vi "sub vi - Read Analog All v9.5.vi"(0 "data 0":waveform(dbl)[](array[waveform]), 5 "data 1":waveform(dbl)[](array[waveform]), 7 "data 2":waveform(dbl)[](array[waveform]), 9 "AI Error":errorcluster[](array[cluster])) -> (3 "array GRAPH":dynamicdata[](array[waveform]), 4 "LAB01":T2, 6 "LAB02":T3, 8 "LAB03":T4, 10 "LAB04":T5, 13 "deg C":dbl, 14 "USB Error":bool[](array[boolean]), 15 "LAB05":T6)   [LabVIEW 2013]
uses:
  program files/Global display 3.vi
  <vilib>/measure/mascope.llb/Amplitude and Levels 1 chan.vi
  <vilib>/addons/Electrical Power/Basic/Measurement/Power (1 Channel).vi
  <vilib>/addons/Electrical Power/Basic/Measurement/RMS (N Channels).vi
  <vilib>/addons/Electrical Power/Basic/Measurement/RMS (1 Channel).vi
  <vilib>/addons/Electrical Power/Basic/NI_EP_Basic.lvlib
  <vilib>/measure/NI_MAPro.lvlib
panel:
  in  "Tab Control":T1(tab)
  out "LAB01-2 (PF)":dbl
  out "LAB01-1 (PF)":dbl
  out "LAB01-2 (V)":dbl
  out "LAB01-2 (A)":dbl
  out "LAB01-1 (V)":dbl
  out "LAB01-1 (A)":dbl
  out "LAB01-2 (GRAPH)":dynamicdata(graph)
  out "LAB01-1 (GRAPH)":dynamicdata(graph)
  out "LAB02-2 (PF)":dbl
  out "LAB02-1 (PF)":dbl
  out "LAB02-2 (V)":dbl
  out "LAB02-2 (A)":dbl
  out "LAB02-1 (V)":dbl
  out "LAB02-1 (A)":dbl
  out "LAB02-2 (GRAPH)":dynamicdata(graph)
  out "LAB02-1 (GRAPH)":dynamicdata(graph)
  out "LAB03-2 (PF)":dbl
  out "LAB03-1 (PF)":dbl
  out "LAB03-2 (V)":dbl
  out "LAB03-2 (A)":dbl
  out "LAB03-1 (V)":dbl
  out "LAB03-1 (A)":dbl
  out "LAB03-2 (GRAPH)":dynamicdata(graph)
  out "LAB03-1 (GRAPH)":dynamicdata(graph)
  out "LAB04-2 (PF)":dbl
  out "LAB04-1 (PF)":dbl
  out "LAB04-2 (V)":dbl
  out "LAB04-2 (A)":dbl
  out "LAB04-1 (V)":dbl
  out "LAB04-1 (A)":dbl
  out "LAB04-1 (GRAPH)":dynamicdata(graph)
  out "LAB04-2 (GRAPH)":dynamicdata(graph)
  out "LAB05-2 (PF)":dbl
  out "LAB05-1 (PF)":dbl
  out "LAB05-2 (V)":dbl
  out "LAB05-2 (A)":dbl
  out "LAB05-1 (V)":dbl
  out "LAB05-1 (A)":dbl
  out "LAB05-1 (GRAPH)":dynamicdata(graph)
  out "LAB05-2 (GRAPH)":dynamicdata(graph)
  out "A1 error":errorcluster
  out "array ERROR":errorcluster[](array[cluster])
  out "AI2-OFF":waveform(dbl)[](graph)
  out "AI2-ON":waveform(dbl)[](graph)
  out "AI1-OFF":waveform(dbl)[](graph)
  out "AI1-ON":waveform(dbl)[](graph)
  out "AI0-OFF":waveform(dbl)[](graph)
  out "AI0-ON":waveform(dbl)[](graph)
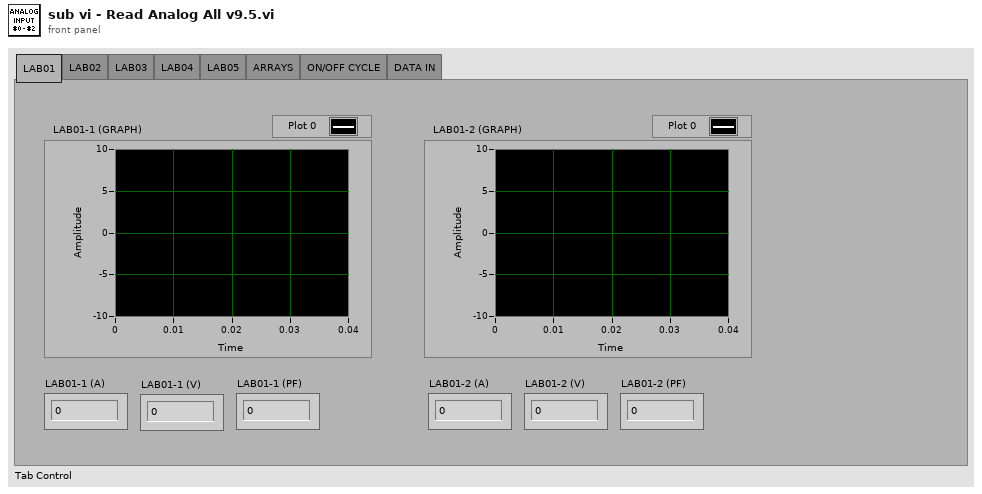
[diagram p1: front panel]
types:
  T1 = enum32{"LAB01", "LAB02", "LAB03", "LAB04", "LAB05", "ARRAYS", "ON/OFF CYCLE", "DATA IN"}
  T2 = cluster{"LAB01-1 (A)":dbl, "LAB01-1 (V)":dbl, "LAB01-1 (PF)":dbl, "LAB01-2 (A)":dbl, "LAB01-2 (V)":dbl, "LAB01-2 (PF)":dbl}
  T3 = cluster{"LAB02-1 (A)":dbl, "LAB02-1 (V)":dbl, "LAB02-1 (PF)":dbl, "LAB02-2 (A)":dbl, "LAB02-2 (V)":dbl, "LAB02-2 (PF)":dbl}
  T4 = cluster{"LAB03-1 (A)":dbl, "LAB03-1 (V)":dbl, "LAB03-1 (PF)":dbl, "LAB03-2 (A)":dbl, "LAB03-2 (V)":dbl, "LAB03-2 (PF)":dbl}
  T5 = cluster{"LAB04-1 (A)":dbl, "LAB04-1 (V)":dbl, "LAB04-1 (PF)":dbl, "LAB04-2 (A)":dbl, "LAB04-2 (V)":dbl, "LAB04-2 (PF)":dbl}
  T6 = cluster{"LAB05-1 (A)":dbl, "LAB05-1 (V)":dbl, "LAB05-1 (PF)":dbl, "LAB05-2 (A)":dbl, "LAB05-2 (V)":dbl, "LAB05-2 (PF)":dbl}
  T7 = typedef "NI_EP_Basic.lvlib/basic_Power Value.ctl" = cluster{"active power [W]":dbl, "apparent power [VA]":dbl, "reactive power [VAR]":dbl, "power factor":dbl}
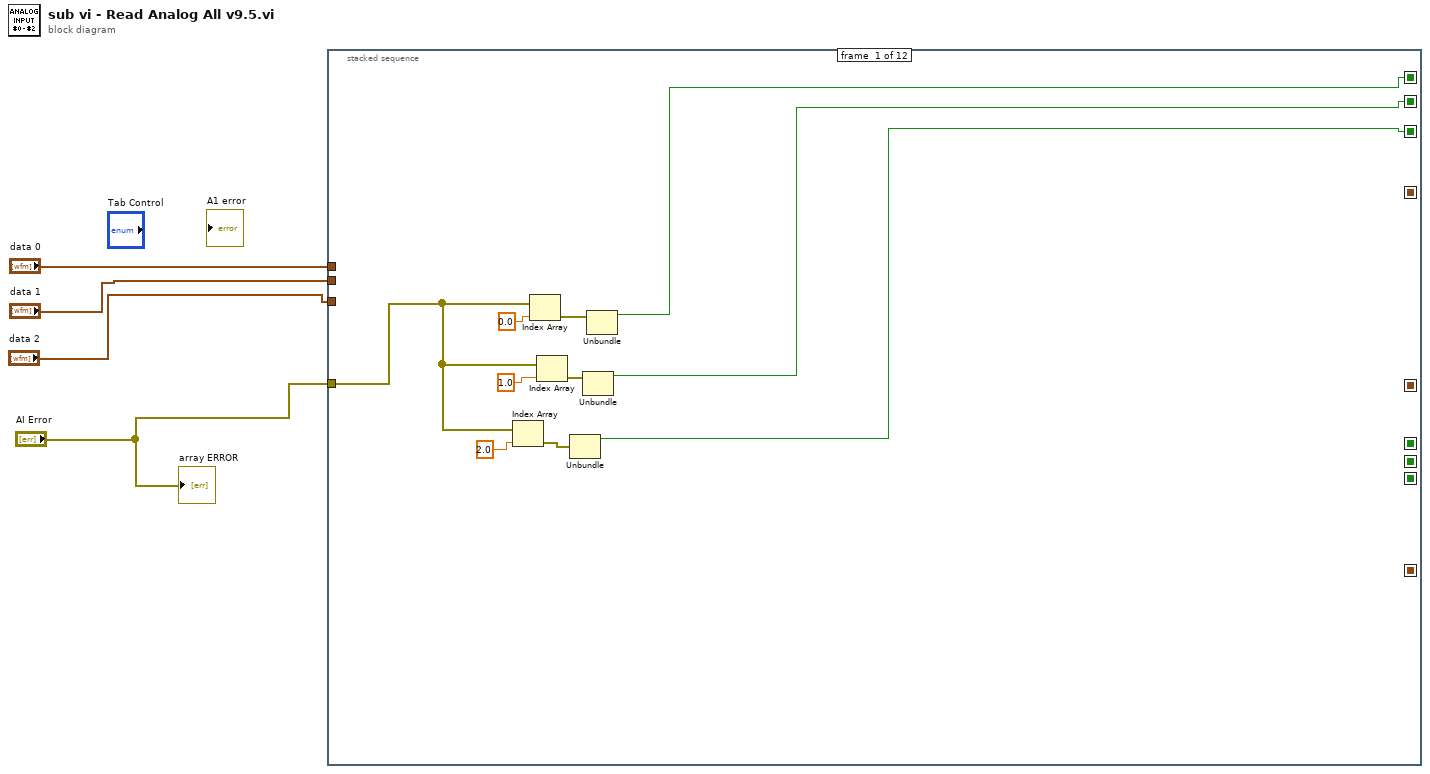
[diagram p0: block diagram]
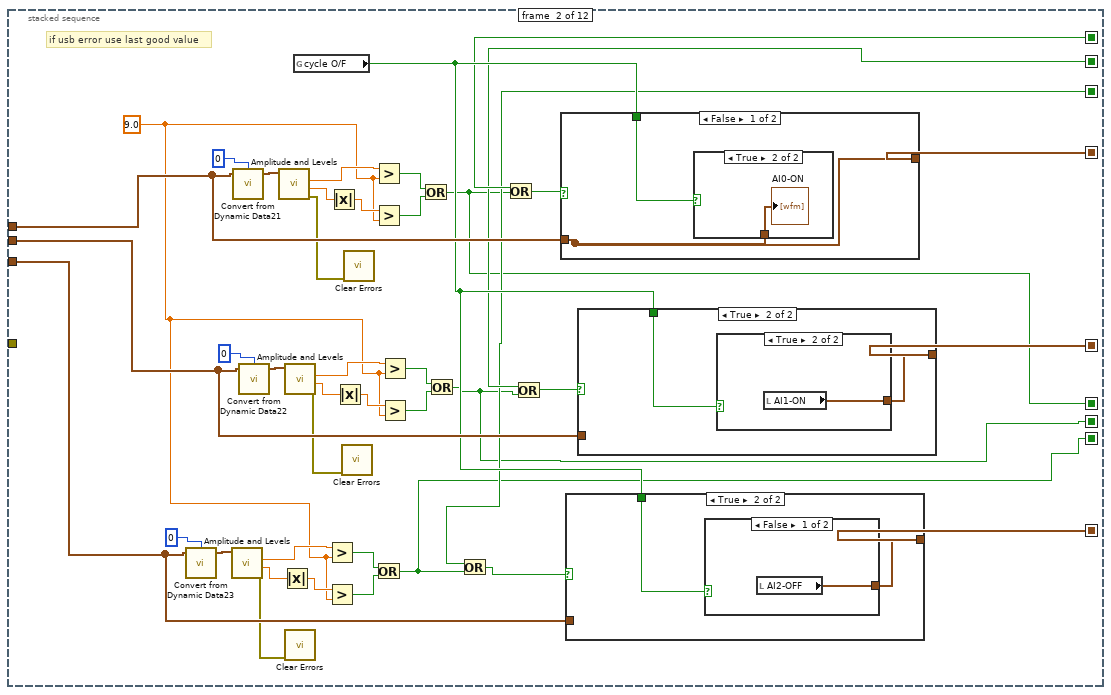
[diagram p2: hidden frame]
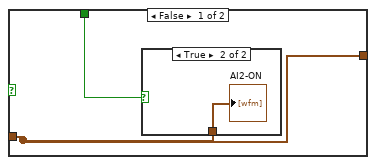
[diagram p3: hidden frame]
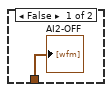
[diagram p4: hidden frame]
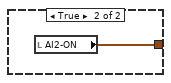
[diagram p5: hidden frame]
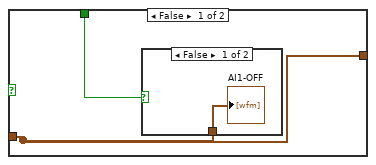
[diagram p6: hidden frame]
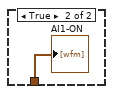
[diagram p7: hidden frame]
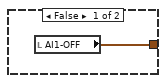
[diagram p8: hidden frame]
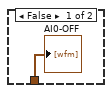
[diagram p9: hidden frame]
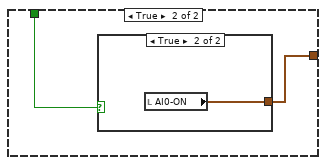
[diagram p10: hidden frame]
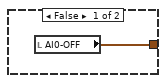
[diagram p11: hidden frame]
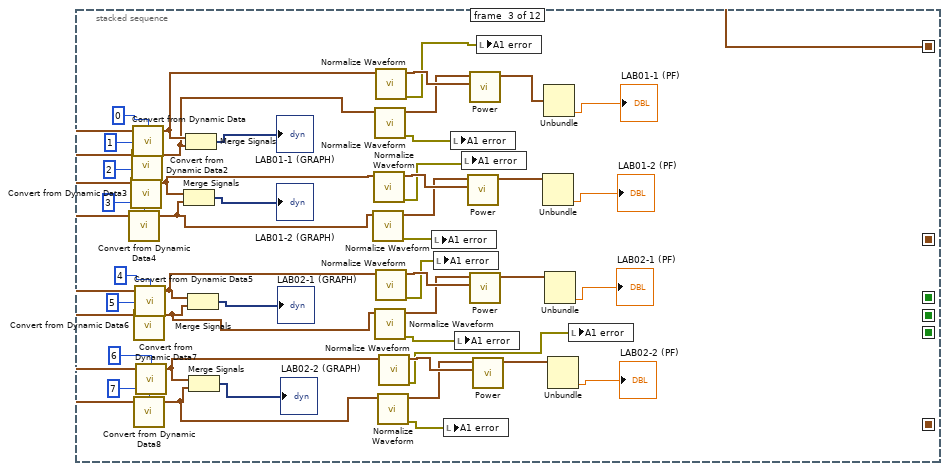
[diagram p12: hidden frame]
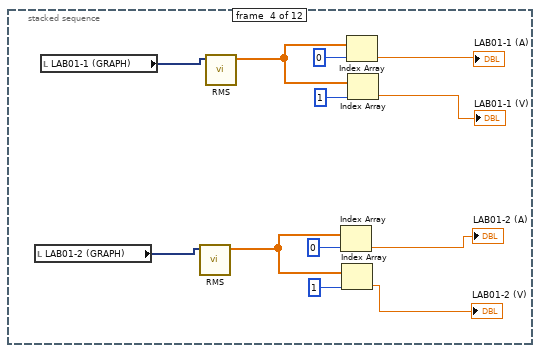
[diagram p13: hidden frame]
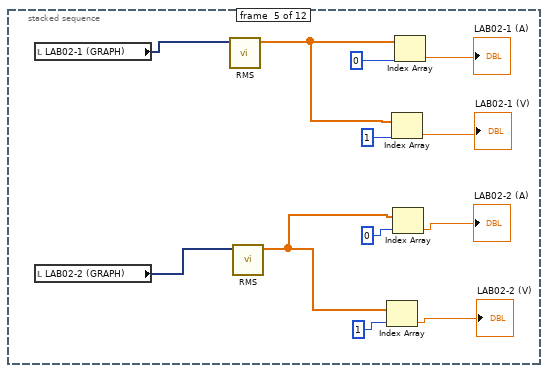
[diagram p14: hidden frame]
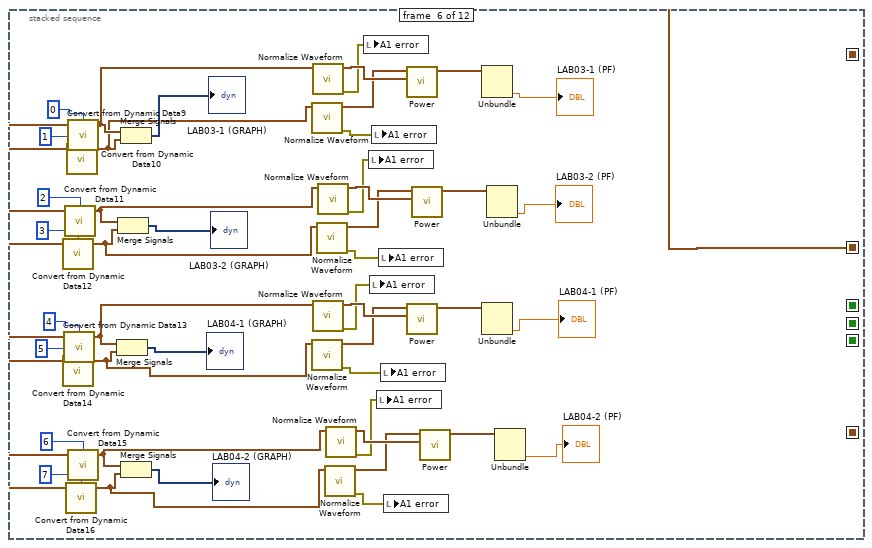
[diagram p15: hidden frame]
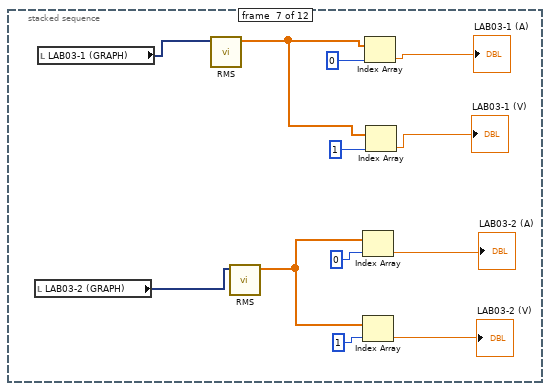
[diagram p16: hidden frame]
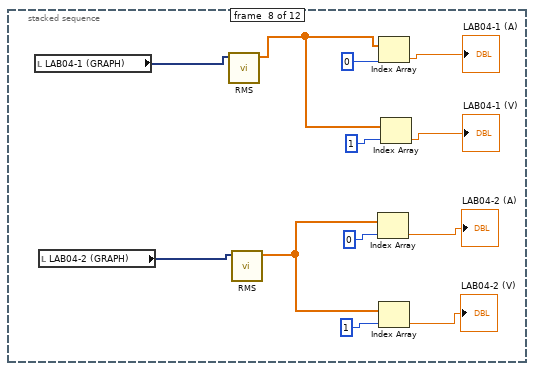
[diagram p17: hidden frame]
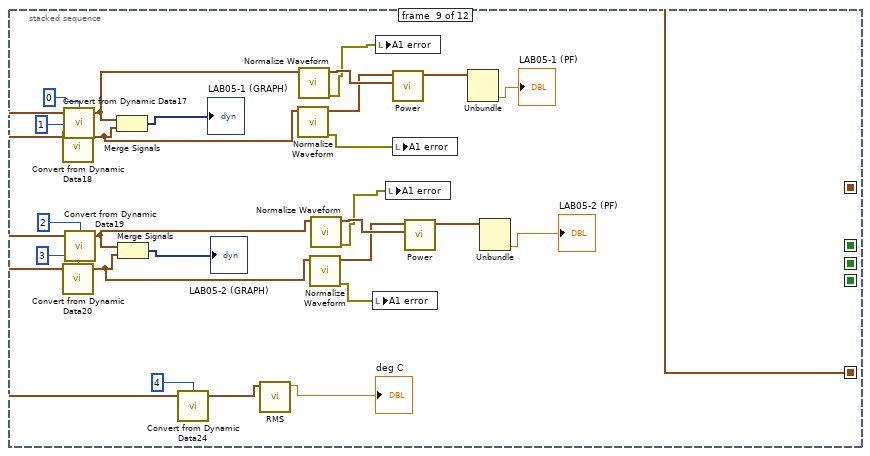
[diagram p18: hidden frame]
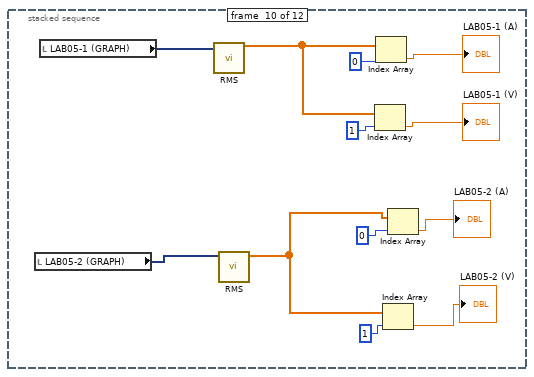
[diagram p19: hidden frame]
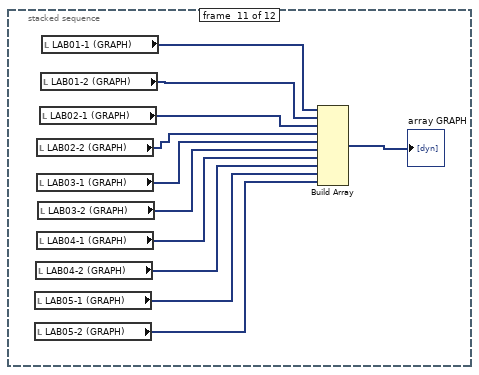
[diagram p20: hidden frame]
diagram:
  n1 = stacked-sequence {
    seq-local: [w12 _ _ _ _ _ _ _ _ _ _ _] -> [_ w22 _ _ _ _ _ _ _ _ _ w272]
    seq-local: [w9 _ _ _ _ _ _ _ _ _ _ _] -> [_ w21 _ _ _ _ _ _ _ _ _ w271]
    seq-local: [w5 _ _ _ _ _ _ _ _ _ _ _] -> [_ w18 _ _ _ _ _ _ _ _ _ w270]
    seq-local: [_ w48 _ _ _ _ _ _ _ _ _ _] -> [_ _ w124 _ _ _ _ _ _ _ _ _]
    seq-local: [_ w38 _ _ _ _ _ _ _ _ _ _] -> [_ _ _ _ _ w193 _ _ _ _ _ _]
    seq-local: [_ w27 _ _ _ _ _ _ _ _ _ _] -> [_ _ _ _ _ _ _ _ w243 _ _ _]
    seq-local: [_ w17 _ _ _ _ _ _ _ _ _ _] -> [_ _ _ _ _ _ _ _ _ _ _ w269]
    seq-local: [_ w16 _ _ _ _ _ _ _ _ _ _] -> [_ _ _ _ _ _ _ _ _ _ _ w268]
    seq-local: [_ w15 _ _ _ _ _ _ _ _ _ _] -> [_ _ _ _ _ _ _ _ _ _ _ w267]
    tunnel: "data 0" -> [_ w47 _ _ _ _ _ _ _ _ _ _]
    tunnel: "data 1" -> [_ w39 _ _ _ _ _ _ _ _ _ _]
    tunnel: "data 2" -> [_ w30 _ _ _ _ _ _ _ _ _ _]
    tunnel: "AI Error" -> [w6 _ _ _ _ _ _ _ _ _ _ _]
    frame #0 {
      n2 = Index Array(array=w6, index=2.0) -> (element=w7:errorcluster)
      n3 = Index Array(array=w6, index=0.0) -> (element=w13:errorcluster)
      n4 = Index Array(array=w6, index=1.0) -> (element=w10:errorcluster)
      n5 = Unbundle(w7) -> ("status"=w5:bool)  [unwired: 2 out]
      n6 = Unbundle(w10) -> ("status"=w9:bool)  [unwired: 2 out]
      n7 = Unbundle(w13) -> ("status"=w12:bool)  [unwired: 2 out]
    }
    frame #1 {
      w29 = 9.0
      # "if usb error use last good value"
      n8 = call "Convert from Dynamic Data23"("Dynamic Data Type"=w30, "Channel"=0) -> ("Waveform"=w36:waveform(dbl))  [unwired: 2 in]
      n9 = call-poly <vilib>:"Amplitude and Levels.vi"("signal in"=w36) -> ("error out"=w24:errorcluster, "low state level"=w35:dbl, "high state level"=w34:dbl)  [unwired: 7 in, 1 out]
      n10 = call "Convert from Dynamic Data21"("Dynamic Data Type"=w47, "Channel"=0) -> ("Waveform"=w54:waveform(dbl))  [unwired: 2 in]
      n11 = call "Convert from Dynamic Data22"("Dynamic Data Type"=w39, "Channel"=0) -> ("Waveform"=w45:waveform(dbl))  [unwired: 2 in]
      n12 = call-poly <vilib>:"Amplitude and Levels.vi"("signal in"=w54) -> ("error out"=w26:errorcluster, "low state level"=w53:dbl, "high state level"=w52:dbl)  [unwired: 7 in, 1 out]
      n13 = Absolute Value(x=w35) -> (abs(x)=w33:dbl)
      n14 = call-poly <vilib>:"Amplitude and Levels.vi"("signal in"=w45) -> ("error out"=w25:errorcluster, "low state level"=w44:dbl, "high state level"=w43:dbl)  [unwired: 7 in, 1 out]
      n15 = call <vilib>:"Clear Errors.vi"("error in (no error)"=w24) -> ()  [unwired: 6 in, 1 out]
      n16 = global read "Global display 3.vi" "cycle O/F"() -> (w28:bool)
      n17 = Greater?(x=w34, y=w29) -> (0:w32:bool)
      n18 = Greater?(x=w33, y=w29) -> (0:w31:bool)
      n19 = Absolute Value(x=w53) -> (abs(x)=w51:dbl)
      n20 = Absolute Value(x=w44) -> (abs(x)=w42:dbl)
      n21 = call <vilib>:"Clear Errors.vi"("error in (no error)"=w25) -> ()  [unwired: 6 in, 1 out]
      n22 = call <vilib>:"Clear Errors.vi"("error in (no error)"=w26) -> ()  [unwired: 6 in, 1 out]
      n23 = Greater?(x=w52, y=w29) -> (0:w50:bool)
      n24 = Greater?(x=w51, y=w29) -> (0:w49:bool)
      n25 = Or(x=w32, y=w31) -> (x .or. y?=w15:bool)
      n26 = Greater?(x=w43, y=w29) -> (0:w41:bool)
      n27 = Greater?(x=w42, y=w29) -> (0:w40:bool)
      n28 = Or(x=w50, y=w49) -> (x .or. y?=w17:bool)
      n29 = Or(x=w41, y=w40) -> (x .or. y?=w16:bool)
      n30 = Or(x=w18, y=w15) -> (x .or. y?=w19:bool)
      n31 = Or(x=w22, y=w17) -> (x .or. y?=w23:bool)
      n32 = Or(x=w21, y=w16) -> (x .or. y?=w20:bool)
      n33 = case shown="False" w23 {
        tunnel: w28 -> [w73 w77]
        tunnel: [w72 w76] -> w48
        tunnel: w47 -> [w72 _]
        frame False {
          n34 = case shown="True" w73 {
            tunnel: w72 -> [w74 w75]
            frame False {
              "AI0-OFF" <- w74
            }
            frame True {
              "AI0-ON" <- w75
            }
          }
        }
        frame True {
          n35 = case shown="True" w77 {
            tunnel: [w78 w79] -> w76
            frame False {
              n36 = local read "AI0-OFF"() -> (w78:waveform(dbl)[])
            }
            frame True {
              n37 = local read "AI0-ON"() -> (w79:waveform(dbl)[])
            }
          }
        }
      }
      n38 = case shown="True" w19 {
        tunnel: w28 -> [w57 w61]
        tunnel: [w56 w60] -> w27
        tunnel: w30 -> [w56 _]
        frame False {
          n39 = case shown="True" w57 {
            tunnel: w56 -> [w58 w59]
            frame False {
              "AI2-OFF" <- w58
            }
            frame True {
              "AI2-ON" <- w59
            }
          }
        }
        frame True {
          n40 = case shown="False" w61 {
            tunnel: [w62 w63] -> w60
            frame False {
              n41 = local read "AI2-OFF"() -> (w62:waveform(dbl)[])
            }
            frame True {
              n42 = local read "AI2-ON"() -> (w63:waveform(dbl)[])
            }
          }
        }
      }
      n43 = case shown="True" w20 {
        tunnel: w28 -> [w65 w69]
        tunnel: [w64 w68] -> w38
        tunnel: w39 -> [w64 _]
        frame False {
          n44 = case shown="False" w65 {
            tunnel: w64 -> [w66 w67]
            frame False {
              "AI1-OFF" <- w66
            }
            frame True {
              "AI1-ON" <- w67
            }
          }
        }
        frame True {
          n45 = case shown="True" w69 {
            tunnel: [w70 w71] -> w68
            frame False {
              n46 = local read "AI1-OFF"() -> (w70:waveform(dbl)[])
            }
            frame True {
              n47 = local read "AI1-ON"() -> (w71:waveform(dbl)[])
            }
          }
        }
      }
    }
    frame #2 {
      n48 = call "Convert from Dynamic Data4"("Dynamic Data Type"=w124, "Channel"=3) -> ("Waveform"=w100:waveform(dbl))  [unwired: 2 in]
      n49 = call "Convert from Dynamic Data3"("Dynamic Data Type"=w124, "Channel"=2) -> ("Waveform"=w101:waveform(dbl))  [unwired: 2 in]
      n50 = call "Convert from Dynamic Data2"("Dynamic Data Type"=w124, "Channel"=1) -> ("Waveform"=w110:waveform(dbl))  [unwired: 2 in]
      n51 = call "Convert from Dynamic Data"("Dynamic Data Type"=w124, "Channel"=0) -> ("Waveform"=w111:waveform(dbl))  [unwired: 2 in]
      n52 = call "Convert from Dynamic Data6"("Dynamic Data Type"=w124, "Channel"=5) -> ("Waveform"=w95:waveform(dbl))  [unwired: 2 in]
      n53 = call "Convert from Dynamic Data8"("Dynamic Data Type"=w124, "Channel"=7) -> ("Waveform"=w89:waveform(dbl))  [unwired: 2 in]
      n54 = call "Convert from Dynamic Data5"("Dynamic Data Type"=w124, "Channel"=4) -> ("Waveform"=w96:waveform(dbl))  [unwired: 2 in]
      n55 = call "Convert from Dynamic Data7"("Dynamic Data Type"=w124, "Channel"=6) -> ("Waveform"=w90:waveform(dbl))  [unwired: 2 in]
      n56 = Merge Signals(w101, w100) -> (→"LAB01-2 (GRAPH)":dynamicdata)
      n57 = Merge Signals(w111, w110) -> (→"LAB01-1 (GRAPH)":dynamicdata)
      n58 = Merge Signals(w96, w95) -> (→"LAB02-1 (GRAPH)":dynamicdata)
      n59 = Merge Signals(w90, w89) -> (→"LAB02-2 (GRAPH)":dynamicdata)
      n60 = call <vilib>:"Normalize Waveform.vi"("waveform in"=w100) -> ("error out"=w84:errorcluster, "normalized waveform"=w104:waveform(dbl))  [unwired: 7 in, 2 out]
      n61 = call <vilib>:"Normalize Waveform.vi"("waveform in"=w101) -> ("error out"=w85:errorcluster, "normalized waveform"=w105:waveform(dbl))  [unwired: 7 in, 2 out]
      n62 = call <vilib>:"Normalize Waveform.vi"("waveform in"=w110) -> ("error out"=w86:errorcluster, "normalized waveform"=w108:waveform(dbl))  [unwired: 7 in, 2 out]
      n63 = call <vilib>:"Normalize Waveform.vi"("waveform in"=w95) -> ("error out"=w82:errorcluster, "normalized waveform"=w98:waveform(dbl))  [unwired: 7 in, 2 out]
      n64 = call <vilib>:"Normalize Waveform.vi"("waveform in"=w111) -> ("error out"=w87:errorcluster, "normalized waveform"=w109:waveform(dbl))  [unwired: 7 in, 2 out]
      n65 = call <vilib>:"Normalize Waveform.vi"("waveform in"=w96) -> ("error out"=w83:errorcluster, "normalized waveform"=w99:waveform(dbl))  [unwired: 7 in, 2 out]
      n66 = call <vilib>:"Normalize Waveform.vi"("waveform in"=w89) -> ("error out"=w80:errorcluster, "normalized waveform"=w92:waveform(dbl))  [unwired: 7 in, 2 out]
      n67 = call <vilib>:"Normalize Waveform.vi"("waveform in"=w90) -> ("error out"=w81:errorcluster, "normalized waveform"=w93:waveform(dbl))  [unwired: 7 in, 2 out]
      n68 = local write "A1 error"(w84) -> ()
      n69 = local write "A1 error"(w83) -> ()
      n70 = local write "A1 error"(w80) -> ()
      n71 = local write "A1 error"(w86) -> ()
      n72 = local write "A1 error"(w82) -> ()
      n73 = local write "A1 error"(w85) -> ()
      n74 = call-poly <vilib>:"Power.vi"("current waveform"=w105, "voltage waveform"=w104) -> ("power value"=w103:T7)  [unwired: 8 in, 1 out]
      n75 = call-poly <vilib>:"Power.vi"("current waveform"=w109, "voltage waveform"=w108) -> ("power value"=w107:T7)  [unwired: 8 in, 1 out]
      n76 = call-poly <vilib>:"Power.vi"("current waveform"=w99, "voltage waveform"=w98) -> ("power value"=w97:T7)  [unwired: 8 in, 1 out]
      n77 = call-poly <vilib>:"Power.vi"("current waveform"=w93, "voltage waveform"=w92) -> ("power value"=w91:T7)  [unwired: 8 in, 1 out]
      n78 = local write "A1 error"(w87) -> ()
      n79 = Unbundle(w103) -> ("power factor"=→"LAB01-2 (PF)":dbl)  [unwired: 3 out]
      n80 = Unbundle(w107) -> ("power factor"=→"LAB01-1 (PF)":dbl)  [unwired: 3 out]
      n81 = Unbundle(w97) -> ("power factor"=→"LAB02-1 (PF)":dbl)  [unwired: 3 out]
      n82 = Unbundle(w91) -> ("power factor"=→"LAB02-2 (PF)":dbl)  [unwired: 3 out]
      n83 = local write "A1 error"(w81) -> ()
    }
    frame #3 {
      n84 = local read "LAB01-2 (GRAPH)"() -> (w133:dynamicdata)
      n85 = local read "LAB01-1 (GRAPH)"() -> (w127:dynamicdata)
      n86 = call-poly <vilib>:"RMS.vi"("waveforms"=w133) -> ("RMS values"=w132:dbl[])  [unwired: 9 in, 1 out]
      n87 = call-poly <vilib>:"RMS.vi"("waveforms"=w127) -> ("RMS values"=w136:dbl[])  [unwired: 9 in, 1 out]
      n88 = Index Array(array=w132, index=0) -> (element=→"LAB01-2 (A)":dbl)
      n89 = Index Array(array=w132, index=1) -> (element=→"LAB01-2 (V)":dbl)
      n90 = Index Array(array=w136, index=0) -> (element=→"LAB01-1 (A)":dbl)
      n91 = Index Array(array=w136, index=1) -> (element=→"LAB01-1 (V)":dbl)
    }
    frame #4 {
      n92 = local read "LAB02-1 (GRAPH)"() -> (w144:dynamicdata)
      n93 = local read "LAB02-2 (GRAPH)"() -> (w140:dynamicdata)
      n94 = call-poly <vilib>:"RMS.vi"("waveforms"=w144) -> ("RMS values"=w143:dbl[])  [unwired: 9 in, 1 out]
      n95 = call-poly <vilib>:"RMS.vi"("waveforms"=w140) -> ("RMS values"=w139:dbl[])  [unwired: 9 in, 1 out]
      n96 = Index Array(array=w139, index=1) -> (element=→"LAB02-2 (V)":dbl)
      n97 = Index Array(array=w143, index=1) -> (element=→"LAB02-1 (V)":dbl)
      n98 = Index Array(array=w139, index=0) -> (element=→"LAB02-2 (A)":dbl)
      n99 = Index Array(array=w143, index=0) -> (element=→"LAB02-1 (A)":dbl)
    }
    frame #5 {
      n100 = call "Convert from Dynamic Data12"("Dynamic Data Type"=w193, "Channel"=3) -> ("Waveform"=w170:waveform(dbl))  [unwired: 2 in]
      n101 = call "Convert from Dynamic Data14"("Dynamic Data Type"=w193, "Channel"=5) -> ("Waveform"=w164:waveform(dbl))  [unwired: 2 in]
      n102 = call "Convert from Dynamic Data13"("Dynamic Data Type"=w193, "Channel"=4) -> ("Waveform"=w165:waveform(dbl))  [unwired: 2 in]
      n103 = call "Convert from Dynamic Data11"("Dynamic Data Type"=w193, "Channel"=2) -> ("Waveform"=w171:waveform(dbl))  [unwired: 2 in]
      n104 = call "Convert from Dynamic Data16"("Dynamic Data Type"=w193, "Channel"=7) -> ("Waveform"=w158:waveform(dbl))  [unwired: 2 in]
      n105 = call "Convert from Dynamic Data10"("Dynamic Data Type"=w193, "Channel"=1) -> ("Waveform"=w176:waveform(dbl))  [unwired: 2 in]
      n106 = call "Convert from Dynamic Data9"("Dynamic Data Type"=w193, "Channel"=0) -> ("Waveform"=w177:waveform(dbl))  [unwired: 2 in]
      n107 = call "Convert from Dynamic Data15"("Dynamic Data Type"=w193, "Channel"=6) -> ("Waveform"=w159:waveform(dbl))  [unwired: 2 in]
      n108 = Merge Signals(w165, w164) -> (→"LAB04-1 (GRAPH)":dynamicdata)
      n109 = Merge Signals(w171, w170) -> (→"LAB03-2 (GRAPH)":dynamicdata)
      n110 = Merge Signals(w177, w176) -> (→"LAB03-1 (GRAPH)":dynamicdata)
      n111 = Merge Signals(w159, w158) -> (→"LAB04-2 (GRAPH)":dynamicdata)
      n112 = call <vilib>:"Normalize Waveform.vi"("waveform in"=w176) -> ("error out"=w155:errorcluster, "normalized waveform"=w179:waveform(dbl))  [unwired: 7 in, 2 out]
      n113 = call <vilib>:"Normalize Waveform.vi"("waveform in"=w164) -> ("error out"=w151:errorcluster, "normalized waveform"=w167:waveform(dbl))  [unwired: 7 in, 2 out]
      n114 = call <vilib>:"Normalize Waveform.vi"("waveform in"=w177) -> ("error out"=w156:errorcluster, "normalized waveform"=w180:waveform(dbl))  [unwired: 7 in, 2 out]
      n115 = call <vilib>:"Normalize Waveform.vi"("waveform in"=w165) -> ("error out"=w152:errorcluster, "normalized waveform"=w168:waveform(dbl))  [unwired: 7 in, 2 out]
      n116 = call <vilib>:"Normalize Waveform.vi"("waveform in"=w170) -> ("error out"=w153:errorcluster, "normalized waveform"=w173:waveform(dbl))  [unwired: 7 in, 2 out]
      n117 = call <vilib>:"Normalize Waveform.vi"("waveform in"=w171) -> ("error out"=w154:errorcluster, "normalized waveform"=w174:waveform(dbl))  [unwired: 7 in, 2 out]
      n118 = call <vilib>:"Normalize Waveform.vi"("waveform in"=w158) -> ("error out"=w149:errorcluster, "normalized waveform"=w161:waveform(dbl))  [unwired: 7 in, 2 out]
      n119 = call <vilib>:"Normalize Waveform.vi"("waveform in"=w159) -> ("error out"=w150:errorcluster, "normalized waveform"=w162:waveform(dbl))  [unwired: 7 in, 2 out]
      n120 = local write "A1 error"(w156) -> ()
      n121 = local write "A1 error"(w154) -> ()
      n122 = local write "A1 error"(w152) -> ()
      n123 = local write "A1 error"(w155) -> ()
      n124 = local write "A1 error"(w150) -> ()
      n125 = local write "A1 error"(w153) -> ()
      n126 = local write "A1 error"(w151) -> ()
      n127 = local write "A1 error"(w149) -> ()
      n128 = call-poly <vilib>:"Power.vi"("current waveform"=w180, "voltage waveform"=w179) -> ("power value"=w178:T7)  [unwired: 8 in, 1 out]
      n129 = call-poly <vilib>:"Power.vi"("current waveform"=w168, "voltage waveform"=w167) -> ("power value"=w166:T7)  [unwired: 8 in, 1 out]
      n130 = call-poly <vilib>:"Power.vi"("current waveform"=w174, "voltage waveform"=w173) -> ("power value"=w172:T7)  [unwired: 8 in, 1 out]
      n131 = call-poly <vilib>:"Power.vi"("current waveform"=w162, "voltage waveform"=w161) -> ("power value"=w160:T7)  [unwired: 8 in, 1 out]
      n132 = Unbundle(w178) -> ("power factor"=→"LAB03-1 (PF)":dbl)  [unwired: 3 out]
      n133 = Unbundle(w166) -> ("power factor"=→"LAB04-1 (PF)":dbl)  [unwired: 3 out]
      n134 = Unbundle(w172) -> ("power factor"=→"LAB03-2 (PF)":dbl)  [unwired: 3 out]
      n135 = Unbundle(w160) -> ("power factor"=→"LAB04-2 (PF)":dbl)  [unwired: 3 out]
    }
    frame #6 {
      n136 = local read "LAB03-2 (GRAPH)"() -> (w200:dynamicdata)
      n137 = local read "LAB03-1 (GRAPH)"() -> (w201:dynamicdata)
      n138 = call-poly <vilib>:"RMS.vi"("waveforms"=w201) -> ("RMS values"=w199:dbl[])  [unwired: 9 in, 1 out]
      n139 = call-poly <vilib>:"RMS.vi"("waveforms"=w200) -> ("RMS values"=w196:dbl[])  [unwired: 9 in, 1 out]
      n140 = Index Array(array=w196, index=0) -> (element=→"LAB03-2 (A)":dbl)
      n141 = Index Array(array=w196, index=1) -> (element=→"LAB03-2 (V)":dbl)
      n142 = Index Array(array=w199, index=0) -> (element=→"LAB03-1 (A)":dbl)
      n143 = Index Array(array=w199, index=1) -> (element=→"LAB03-1 (V)":dbl)
    }
    frame #7 {
      n144 = local read "LAB04-1 (GRAPH)"() -> (w213:dynamicdata)
      n145 = local read "LAB04-2 (GRAPH)"() -> (w209:dynamicdata)
      n146 = call-poly <vilib>:"RMS.vi"("waveforms"=w213) -> ("RMS values"=w212:dbl[])  [unwired: 9 in, 1 out]
      n147 = call-poly <vilib>:"RMS.vi"("waveforms"=w209) -> ("RMS values"=w208:dbl[])  [unwired: 9 in, 1 out]
      n148 = Index Array(array=w208, index=0) -> (element=→"LAB04-2 (A)":dbl)
      n149 = Index Array(array=w212, index=0) -> (element=→"LAB04-1 (A)":dbl)
      n150 = Index Array(array=w208, index=1) -> (element=→"LAB04-2 (V)":dbl)
      n151 = Index Array(array=w212, index=1) -> (element=→"LAB04-1 (V)":dbl)
    }
    frame #8 {
      n152 = call "Convert from Dynamic Data18"("Dynamic Data Type"=w243, "Channel"=1) -> ("Waveform"=w232:waveform(dbl))  [unwired: 2 in]
      n153 = call "Convert from Dynamic Data20"("Dynamic Data Type"=w243, "Channel"=3) -> ("Waveform"=w226:waveform(dbl))  [unwired: 2 in]
      n154 = call "Convert from Dynamic Data17"("Dynamic Data Type"=w243, "Channel"=0) -> ("Waveform"=w233:waveform(dbl))  [unwired: 2 in]
      n155 = call "Convert from Dynamic Data19"("Dynamic Data Type"=w243, "Channel"=2) -> ("Waveform"=w227:waveform(dbl))  [unwired: 2 in]
      n156 = Merge Signals(w233, w232) -> (→"LAB05-1 (GRAPH)":dynamicdata)
      n157 = Merge Signals(w227, w226) -> (→"LAB05-2 (GRAPH)":dynamicdata)
      n158 = call "Convert from Dynamic Data24"("Dynamic Data Type"=w243, "Channel"=4) -> ("Waveform"=w219:waveform(dbl))  [unwired: 2 in]
      n159 = call-poly <vilib>:"RMS.vi"("waveform"=w219) -> ("RMS value"=→"deg C":dbl)  [unwired: 9 in, 1 out]
      n160 = call <vilib>:"Normalize Waveform.vi"("waveform in"=w232) -> ("error out"=w224:errorcluster, "normalized waveform"=w235:waveform(dbl))  [unwired: 7 in, 2 out]
      n161 = call <vilib>:"Normalize Waveform.vi"("waveform in"=w233) -> ("error out"=w223:errorcluster, "normalized waveform"=w236:waveform(dbl))  [unwired: 7 in, 2 out]
      n162 = call <vilib>:"Normalize Waveform.vi"("waveform in"=w226) -> ("error out"=w222:errorcluster, "normalized waveform"=w229:waveform(dbl))  [unwired: 7 in, 2 out]
      n163 = call <vilib>:"Normalize Waveform.vi"("waveform in"=w227) -> ("error out"=w221:errorcluster, "normalized waveform"=w230:waveform(dbl))  [unwired: 7 in, 2 out]
      n164 = local write "A1 error"(w222) -> ()
      n165 = local write "A1 error"(w223) -> ()
      n166 = local write "A1 error"(w221) -> ()
      n167 = call-poly <vilib>:"Power.vi"("current waveform"=w236, "voltage waveform"=w235) -> ("power value"=w234:T7)  [unwired: 8 in, 1 out]
      n168 = local write "A1 error"(w224) -> ()
      n169 = call-poly <vilib>:"Power.vi"("current waveform"=w230, "voltage waveform"=w229) -> ("power value"=w228:T7)  [unwired: 8 in, 1 out]
      n170 = Unbundle(w234) -> ("power factor"=→"LAB05-1 (PF)":dbl)  [unwired: 3 out]
      n171 = Unbundle(w228) -> ("power factor"=→"LAB05-2 (PF)":dbl)  [unwired: 3 out]
    }
    frame #9 {
      n172 = local read "LAB05-2 (GRAPH)"() -> (w250:dynamicdata)
      n173 = local read "LAB05-1 (GRAPH)"() -> (w251:dynamicdata)
      n174 = call-poly <vilib>:"RMS.vi"("waveforms"=w251) -> ("RMS values"=w249:dbl[])  [unwired: 9 in, 1 out]
      n175 = call-poly <vilib>:"RMS.vi"("waveforms"=w250) -> ("RMS values"=w248:dbl[])  [unwired: 9 in, 1 out]
      n176 = Index Array(array=w249, index=1) -> (element=→"LAB05-1 (V)":dbl)
      n177 = Index Array(array=w249, index=0) -> (element=→"LAB05-1 (A)":dbl)
      n178 = Index Array(array=w248, index=1) -> (element=→"LAB05-2 (V)":dbl)
      n179 = Index Array(array=w248, index=0) -> (element=→"LAB05-2 (A)":dbl)
    }
    frame #10 {
      n180 = local read "LAB05-1 (GRAPH)"() -> (w258:dynamicdata)
      n181 = local read "LAB05-2 (GRAPH)"() -> (w257:dynamicdata)
      n182 = local read "LAB04-2 (GRAPH)"() -> (w259:dynamicdata)
      n183 = local read "LAB02-2 (GRAPH)"() -> (w263:dynamicdata)
      n184 = local read "LAB03-1 (GRAPH)"() -> (w262:dynamicdata)
      n185 = local read "LAB04-1 (GRAPH)"() -> (w260:dynamicdata)
      n186 = local read "LAB03-2 (GRAPH)"() -> (w261:dynamicdata)
      n187 = local read "LAB02-1 (GRAPH)"() -> (w264:dynamicdata)
      n188 = local read "LAB01-2 (GRAPH)"() -> (w265:dynamicdata)
      n189 = local read "LAB01-1 (GRAPH)"() -> (w266:dynamicdata)
      n190 = Build Array(w266, w265, w264, w263, w262, w261, w260, w259, w258, w257) -> (→"array GRAPH":dynamicdata[])
    }
    frame #11 {
      n191 = local read "LAB03-2 (PF)"() -> (w291:dbl)
      n192 = local read "LAB03-1 (PF)"() -> (w294:dbl)
      n193 = local read "LAB03-1 (A)"() -> (w296:dbl)
      n194 = local read "LAB03-1 (V)"() -> (w295:dbl)
      n195 = local read "LAB03-2 (A)"() -> (w293:dbl)
      n196 = local read "LAB03-2 (V)"() -> (w292:dbl)
      n197 = local read "LAB01-1 (PF)"() -> (w301:dbl)
      n198 = local read "LAB01-2 (PF)"() -> (w298:dbl)
      n199 = local read "LAB01-1 (V)"() -> (w302:dbl)
      n200 = local read "LAB01-2 (A)"() -> (w300:dbl)
      n201 = local read "LAB01-2 (V)"() -> (w299:dbl)
      n202 = local read "LAB01-1 (A)"() -> (w303:dbl)
      n203 = Bundle("LAB03-1 (A)"=w296, "LAB03-1 (V)"=w295, "LAB03-1 (PF)"=w294, "LAB03-2 (A)"=w293, "LAB03-2 (V)"=w292, "LAB03-2 (PF)"=w291) -> (→"LAB03":T4)  [unwired: 1 in]
      n204 = local read "LAB05-2 (PF)"() -> (w277:dbl)
      n205 = local read "LAB05-1 (PF)"() -> (w280:dbl)
      n206 = Bundle("LAB01-1 (A)"=w303, "LAB01-1 (V)"=w302, "LAB01-1 (PF)"=w301, "LAB01-2 (A)"=w300, "LAB01-2 (V)"=w299, "LAB01-2 (PF)"=w298) -> (→"LAB01":T2)  [unwired: 1 in]
      n207 = local read "LAB05-2 (V)"() -> (w278:dbl)
      n208 = local read "LAB05-1 (A)"() -> (w282:dbl)
      n209 = local read "LAB05-1 (V)"() -> (w281:dbl)
      n210 = local read "LAB05-2 (A)"() -> (w279:dbl)
      n211 = local read "LAB04-1 (PF)"() -> (w288:dbl)
      n212 = local read "LAB04-2 (PF)"() -> (w285:dbl)
      n213 = local read "LAB04-1 (A)"() -> (w290:dbl)
      n214 = local read "LAB04-1 (V)"() -> (w289:dbl)
      n215 = local read "LAB04-2 (A)"() -> (w287:dbl)
      n216 = local read "LAB04-2 (V)"() -> (w286:dbl)
      n217 = local read "LAB02-2 (PF)"() -> (w305:dbl)
      n218 = local read "LAB02-1 (PF)"() -> (w308:dbl)
      n219 = local read "LAB02-2 (A)"() -> (w307:dbl)
      n220 = local read "LAB02-2 (V)"() -> (w306:dbl)
      n221 = local read "LAB02-1 (V)"() -> (w309:dbl)
      n222 = local read "LAB02-1 (A)"() -> (w310:dbl)
      n223 = Bundle("LAB05-1 (A)"=w282, "LAB05-1 (V)"=w281, "LAB05-1 (PF)"=w280, "LAB05-2 (A)"=w279, "LAB05-2 (V)"=w278, "LAB05-2 (PF)"=w277) -> (→"LAB05":T6)  [unwired: 1 in]
      n224 = Bundle("LAB04-1 (A)"=w290, "LAB04-1 (V)"=w289, "LAB04-1 (PF)"=w288, "LAB04-2 (A)"=w287, "LAB04-2 (V)"=w286, "LAB04-2 (PF)"=w285) -> (→"LAB04":T5)  [unwired: 1 in]
      n225 = Bundle("LAB02-1 (A)"=w310, "LAB02-1 (V)"=w309, "LAB02-1 (PF)"=w308, "LAB02-2 (A)"=w307, "LAB02-2 (V)"=w306, "LAB02-2 (PF)"=w305) -> (→"LAB02":T3)  [unwired: 1 in]
      n226 = Or(x=w271, y=w268) -> (x .or. y?=w273:bool)
      n227 = Or(x=w272, y=w267) -> (x .or. y?=w275:bool)
      n228 = Or(x=w270, y=w269) -> (x .or. y?=w274:bool)
      n229 = Build Array(w275, w273, w274) -> (→"USB Error":bool[])
    }
  }
  "array ERROR" <- "AI Error"
